vi "PathPlanner_Trajectory_ReadCSVFile.vi"(8 "error in (no error)":errorcluster, 11 "FileName":string="trajectory.csv") -> (0 "error out":errorcluster, 3 "outTRAJECTORY":T1 {"States"."TargetHolonomicRotation"."SIN" format="%13.4f"; "States"."TargetHolonomicRotation"."COS" format="%13.4f"; "States"."TargetHolonomicRotation"."VALUE" format="%13.4f"; "States"."Heading"."SIN" format="%13.4f"; "States"."Heading"."COS" format="%13.4f"; "States"."Heading"."VALUE" format="%13.4f"; "States"."PositionMeters"."Y" format="%14.3f"; "States"."PositionMeters"."X" format="%14.3f"}, 4 "Full FIlename":string)   [LabVIEW 2019, in "PathPlanner24.lvlib"]
doc: "Create a trajectory from a CSV file. This can be used on a PC or the RoboRIO. Normally the CSV file is created as output from one of the trajectory utility programs. The file could also be created manually or by a custom written program.\n\nParameters:\n - FileName -- Name of the CSV file to read. See file name notes for additional information.\n - Error In -- Input error cluster (optional)\n\nReturns:\n - outTrajectory - Trajectory data structure cluster\n - Error out - returned error cluster\n\nNotes on use:\n -- This routine writes informational messges to the console and to the driver station log.\n\nNotes on file naming:\n -- The file name must include the extention. \".csv\" is not automatically appended to the name. \n -- The file name can be a simple file or an absolute path. If a simple file name is used the default path on the RoboRIO is: \"home:\\lvuser\\natinst\\LabVIEW Data\". On a Windows PC the default path is the LabVIEW default directory. Normally this is: “%HOMEDRIVE%%HOMEPATH%\\Documents\\LabView Data\".\n -- Filenames on the RoboRIO, which runs Linux, are case sensitive.\n\nNotes on file contents:\n -- Blank lines are ignored.\n -- Lines that begin with either #, !, or ' in the first character are considered comments and are ignored. \n -- Other lines are interpretted as comma separated data as follows:\n -- Trajectory time -- seconds\n -- Expected velocity -- meters/sec\n -- Expected acceleration -- meters/sec^2\n -- Expected X position -- meters\n -- Expected Y position -- meters\n -- Expected heading (not necessarily robot orientation) -- radians\n -- Expected curvature (rotational portion of velocity) -- radians/meter\n -- Optional comment string. This ignored when reading file"
uses:
  PathPlanner24.lvlib
  <vilib>/Utility/error.llb/whitespace.ctl
  <vilib>/Rock Robotics/WPI/ThirdParty/JAS_Junk/TrajLib/TypeDef/TRANSLATION2D.ctl
  <vilib>/Rock Robotics/WPI/ThirdParty/JAS_Junk/TrajLib/Trajectory_Library.lvlib
  <vilib>/Rock Robotics/WPI/ThirdParty/JAS_Junk/TrajLib/TypeDef/ROTATION2D.ctl
  TypeDef/PathPlannerTrajectoryState.ctl
  TypeDef/PathPlannerConstraints.ctl
  TypeDef/PathPlannerTrajectory.ctl
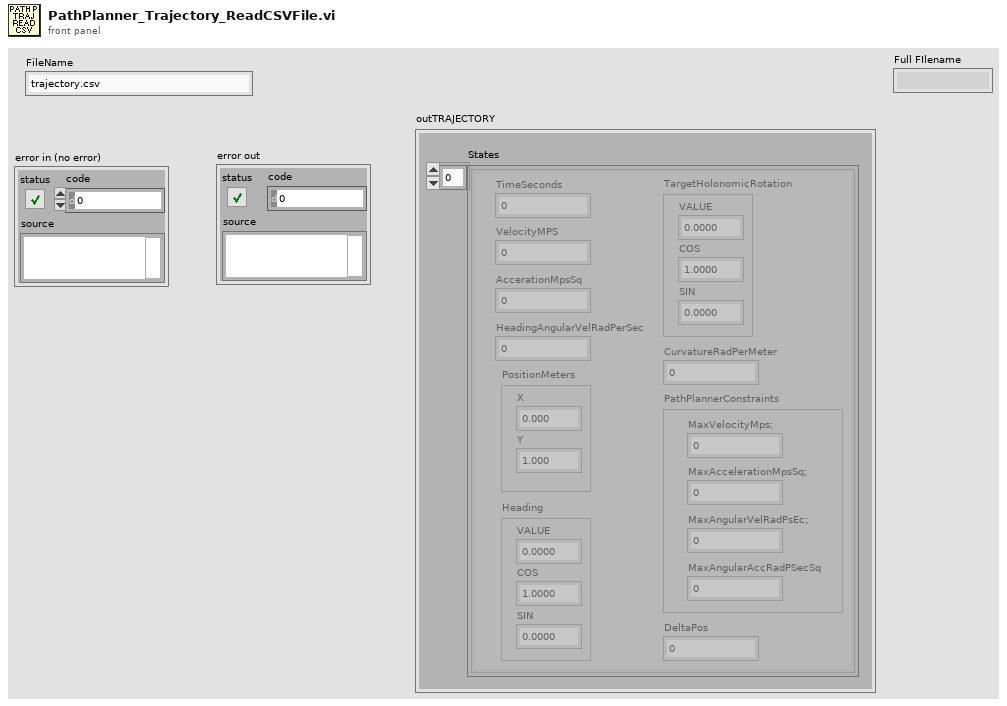
[diagram p1: front panel]
types:
  T1 = typedef "PathPlanner24.lvlib/PathPlannerTrajectory.ctl" = cluster{"States":T2[]}
  T2 = typedef "PathPlanner24.lvlib/PathPlannerTrajectoryState.ctl" = cluster{"TimeSeconds":dbl, "VelocityMPS":dbl, "AccerationMpsSq":dbl, "HeadingAngularVelRadPerSec":dbl, "PositionMeters":T3, "Heading":T4, "TargetHolonomicRotation":T4, "CurvatureRadPerMeter":dbl, "DeltaPos":dbl, "PathPlannerConstraints":T5}
  T3 = typedef "Trajectory_Library.lvlib/TRANSLATION2D.ctl" = cluster{"X":dbl, "Y":dbl}
  T4 = typedef "Trajectory_Library.lvlib/ROTATION2D.ctl" = cluster{"VALUE":dbl, "COS":dbl, "SIN":dbl}
  T5 = typedef "PathPlanner24.lvlib/PathPlannerConstraints.ctl" = cluster{"MaxVelocityMps;":dbl, "MaxAccelerationMpsSq;":dbl, "MaxAngularVelRadPsEc;":dbl, "MaxAngularAccRadPSecSq":dbl}
  T6 = enum16{"open", "replace", "create", "open or create", "replace or create", "replace or create with confirmation"}
  T7 = typedef "whitespace.ctl" = u16
  T8 = typedef "Trajectory_Library.lvlib/POSE2D.ctl" = cluster{"TRANSLATION":T3, "ROTATION":T4}
  T9 = typedef "PathPlanner24.lvlib/PathPlannerTrajectory.ctl" = cluster{"TotalTimeSeconds":dbl, "States":T2[]}
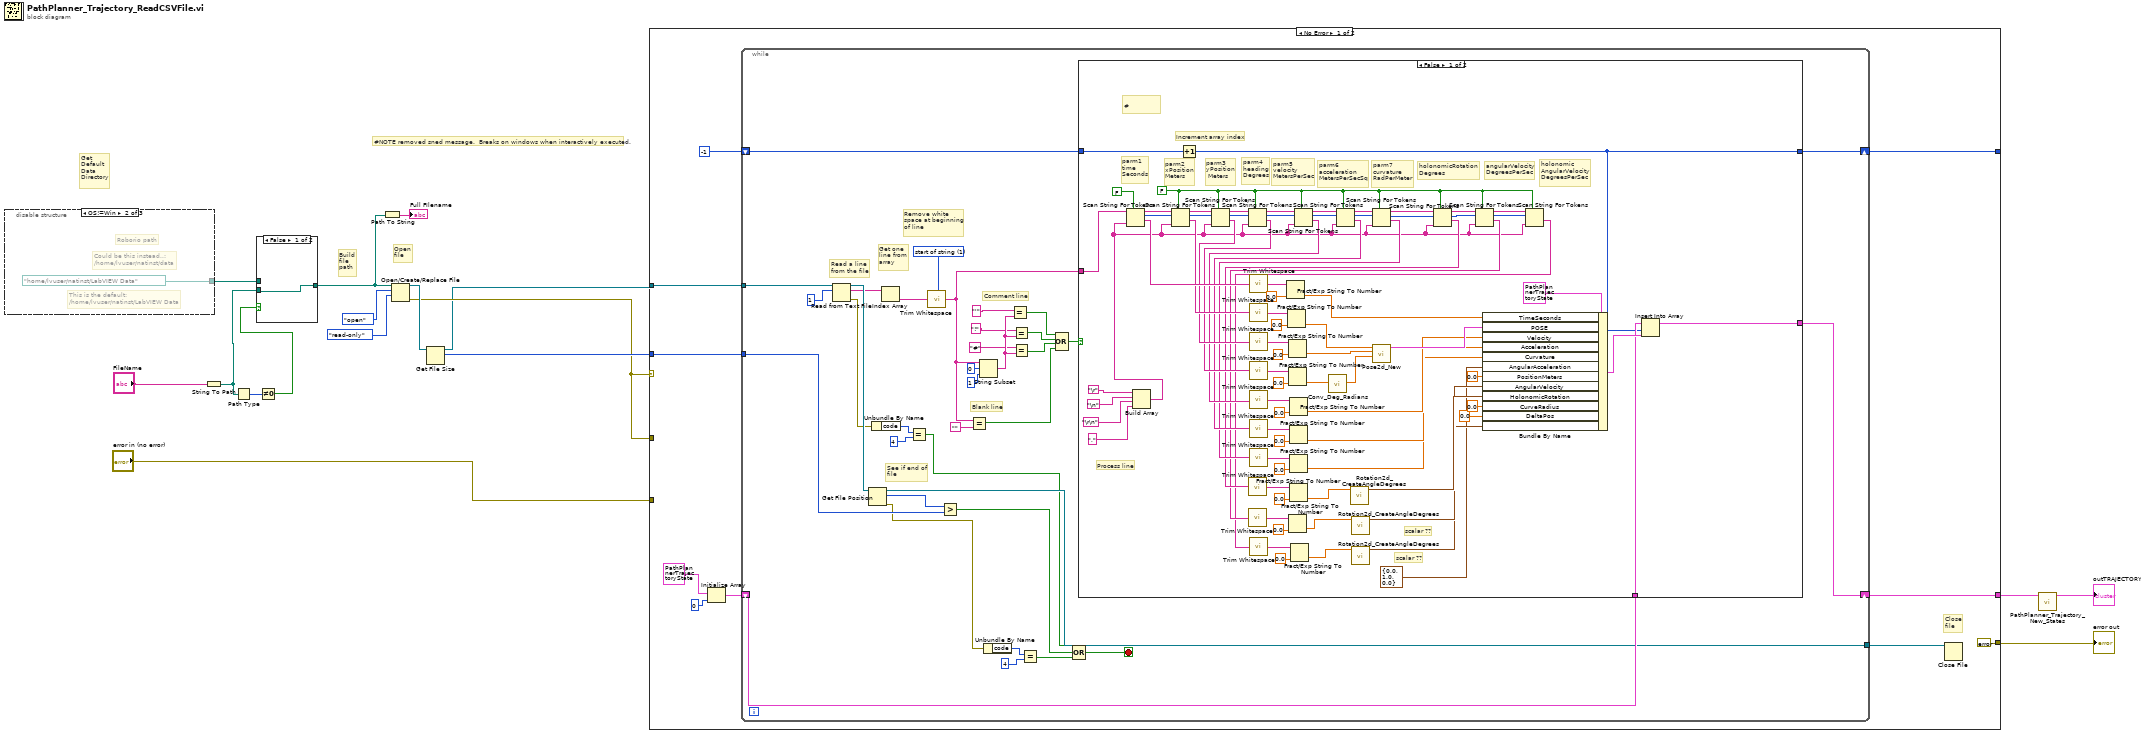
[diagram p0: block diagram]
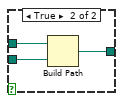
[diagram p2: hidden frame]
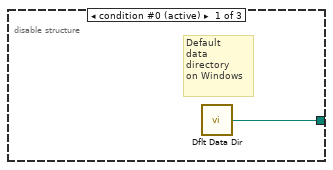
[diagram p3: hidden frame]
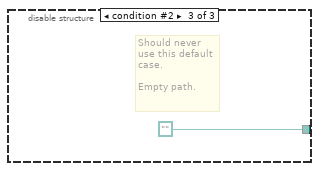
[diagram p4: hidden frame]
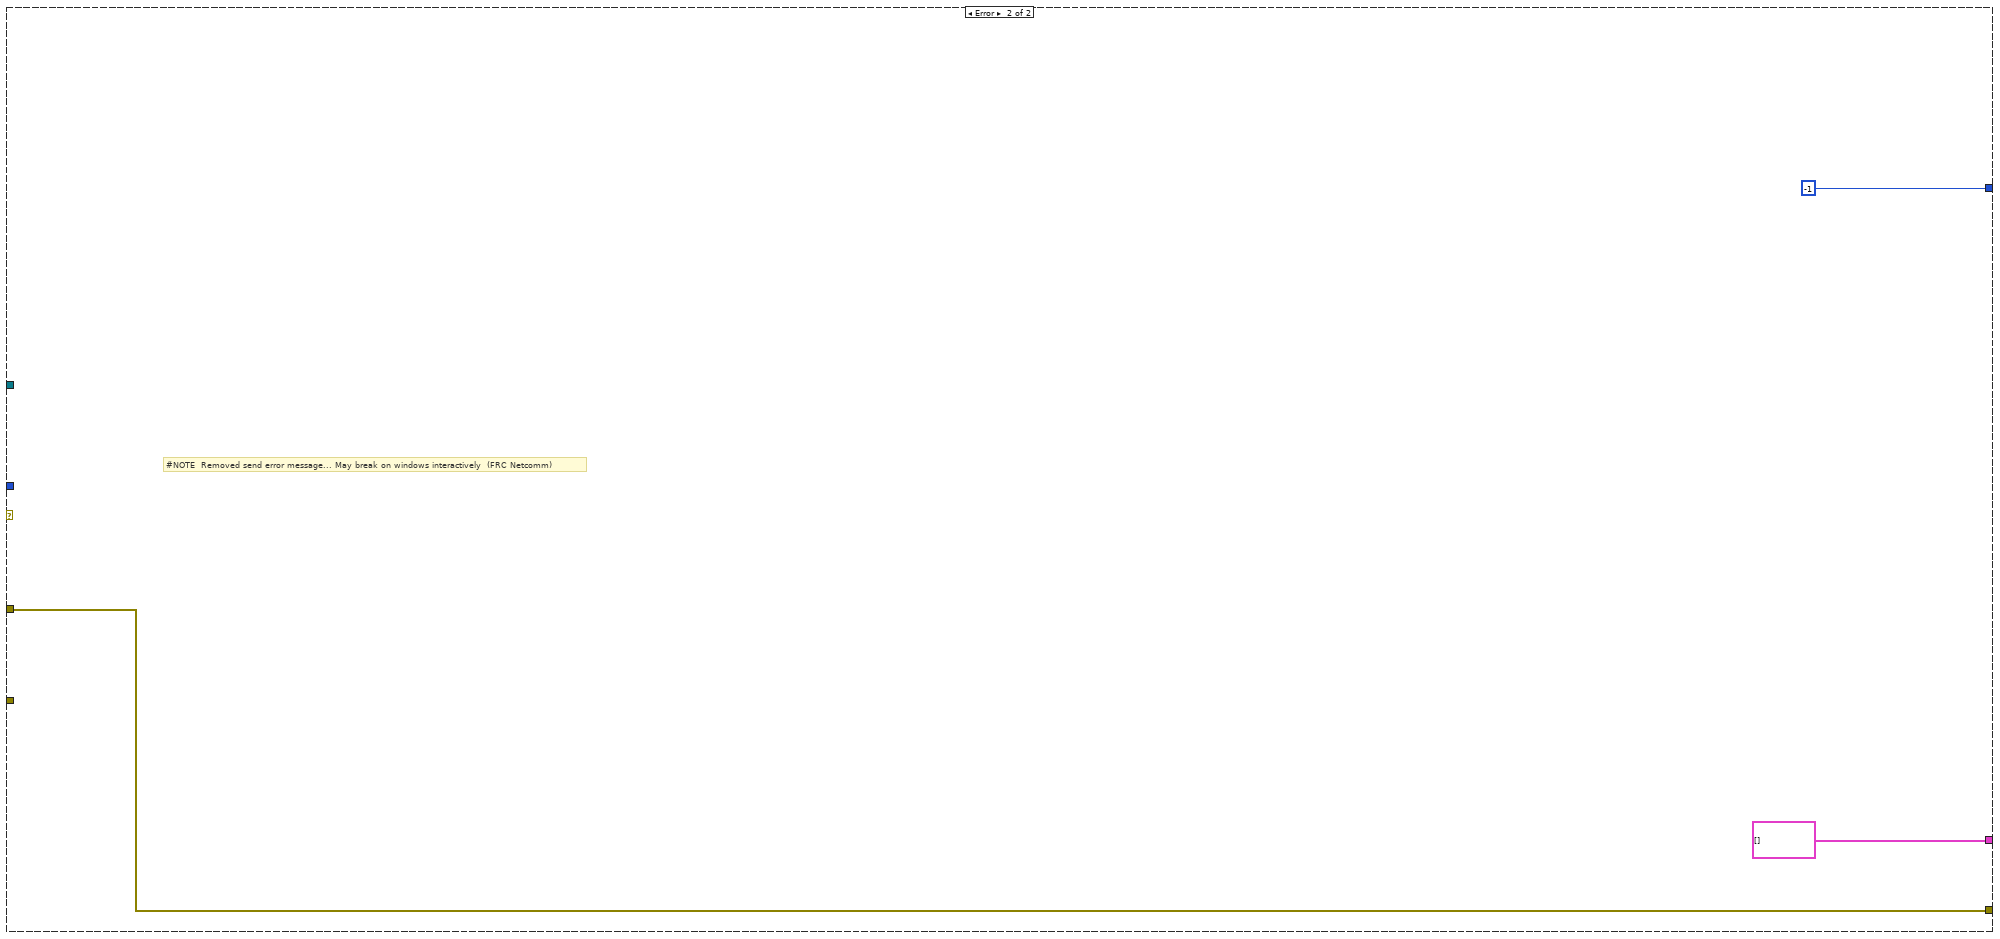
[diagram p6: hidden frame]
diagram:
  # "#NOTE removed sned message.  Breaks on windows when interactively executed."
  # "Get\nDefault\nData\nDirectory"
  # "Open\nfile"
  # "Build\nfile\npath"
  n1 = disable-structure shown="OS!=Win" {
    disable-tunnel: [w18 path "/home/lvuser/natinst/LabVIEW Data" path ""] -> w11
    frame condition #0 (active) {
      # "Default\ndata\ndirectory\non Windows"
      n2 = call <vilib>:"Dflt Data Dir.vi"() -> ("App:Default Data Directory"=w18:path)
    }
    frame condition #1 {
      # "This is the default:\n/home/lvuser/natinst/LabVIEW Data"
      # "Could be this instead..:\n/home/lvuser/natinst/data"
      # "Roborio path"
    }
    frame condition #2 {
      # "Should never\nuse this default\ncase.\n\nEmpty path."
    }
  }
  n3 = String To Path(string="FileName") -> (path=w8:path)
  n4 = Path Type(1:w8) -> (0:w7:i16)
  n5 = Not Equal To 0?(x=w7) -> (x != 0?=w6:bool)
  n6 = case shown="False" w6 {
    tunnel: [w21 w24] -> w14
    tunnel: w11 -> [_ w23]
    tunnel: w8 -> [w21 w22]
    frame False {
    }
    frame True {
      n7 = Build Path(base path=w23, name or relative path=w22) -> (appended path=w24:path)
    }
  }
  n8 = Path To String(path=w14) -> (string=→"Full FIlename":string)
  n9 = Open/Create/Replace File(file path (use dialog)=w14, operation (0:open)=T6."open", access (0:read/write)=enum16{"read/write", "read-only", "write-only"}."read-only") -> (refnum out=w15:refnum<file>, error out=w12:errorcluster)  [unwired: 3 in, 1 out]
  n10 = Get File Size(file=w15) -> (refnum out=w5:refnum<file>, size (in bytes)=w13:i64)  [unwired: 1 in, 1 out]
  n11 = case shown="No Error" w12 {
    tunnel: w5 -> [w34 _]
    tunnel: w13 -> [w32 _]
    tunnel: [w28 i16 -1] -> _
    tunnel: [w27 T2[] []] -> w2
    tunnel: w12 -> [_ w154]
    tunnel: [errorcluster {"status"=FALSE, "code"=0, "source"=""} ("error out") w154] -> w10
    tunnel: "error in (no error)" -> [_ _]
    frame No Error {
      # "Close\nfile"
      n12 = Initialize Array(T2 {"TimeSeconds"=0.0, "VelocityMPS"=0.0, "AccerationMpsSq"=0.0, "HeadingAngularVelRadPerSec"=0.0, "PositionMeters"={"X"=0.0, "Y"=1.0}, "Heading"={"VALUE"=0.0, "COS"=1.0, "SIN"=0.0}, "TargetHolonomicRotation"={"VALUE"=0.0, "COS"=1.0, "SIN"=0.0}, "CurvatureRadPerMeter"=0.0, "DeltaPos"=0.0, "PathPlannerConstraints"={"MaxVelocityMps;"=0.0, "MaxAccelerationMpsSq;"=0.0, "MaxAngularVelRadPsEc;"=0.0, "MaxAngularAccRadPSecSq"=0.0}} ("PathPlannerState"), 0 ("dimension size")) -> (w29:T2[])
      n13 = while {
        tunnel: w34 -> [w70]
        tunnel: w32 -> [w66]
        tunnel: [w46] -> w31
        shift-right: [w36] -> w28
        shift-left: i16 -1 -> [w50]
        shift-right: [w35] -> w27
        shift-left: w29 -> [w48]
        stop <- w44 stop-if-true
        w65 = T7 1 items=["both", "start of string", "end of string"] ("location (both)")
        # "Comment line"
        # "Blank line"
        # "Remove white \nspace at beginning\nof line"
        # "Get one\nline from\narray"
        # "Read a line\nfrom the file"
        # "See if end of \nfile"
        n14 = Read from Text File(file (use dialog)=w70, count=1) -> (refnum out=w68:refnum<file>, text=w64:string[], error out=w47:errorcluster)  [unwired: 2 in, 1 out]
        n15 = Get File Position(7:w68) -> (0:w39:errorcluster, 2:w67:i64, 3:w46:refnum<file>)  [unwired: 1 in]
        n16 = Unbundle By Name(w47) -> ("code"=w43:i32)
        n17 = Index Array(array=w64) -> (element=w63:string)  [unwired: 1 in]
        n18 = Equal?(x=w43, y=4) -> (x = y?=w38:bool)
        n19 = call <vilib>:"Trim Whitespace.vi"("string"=w63, "location (both)"=w65) -> ("trimmed string"=w49:string)
        n20 = Greater?(x=w67, y=w66) -> (0:w45:bool)
        n21 = Equal?(x=w49, y="") -> (x = y?=w52:bool)
        n22 = String Subset(string=w49, offset (0)=0, length (rest)=1 ("length (rest)")) -> (substring=w59:string)
        n23 = Unbundle By Name(w39) -> ("code"=w41:i32)
        n24 = Equal?(x="'", y=w59) -> (x = y?=w55:bool)
        n25 = Equal?(x="!", y=w59) -> (x = y?=w54:bool)
        n26 = Equal?(x="#", y=w59) -> (x = y?=w53:bool)
        n27 = Equal?(x=w41, y=4) -> (x = y?=w37:bool)
        n28 = Compound Arithmetic op=OR(w55, w54, w53, w52) -> (w51:bool)
        n29 = Compound Arithmetic op=OR(w38, w45, w37) -> (w44:bool)
        n30 = case shown="False" w51 {
          tunnel: w50 -> [w151 w152]
          tunnel: [w116 w152] -> w36
          tunnel: w49 -> [w115 _]
          tunnel: w48 -> [w118 w153]
          tunnel: [w117 w153] -> w35
          frame False {
            w97 = FALSE ("allow empty tokens? (F)")
            # "scalar ??"
            # "scalar ??"
            # "holonomic\nAngularVelocity\nDegreesPerSec"
            # "angularVelocity\nDegreesPerSec"
            # "holonomicRotation\nDegrees"
            # "#"
            # "parm6\nacceleration\nMetersPerSecSq"
            # "parm7\ncurvature\nRadPerMeter"
            # "parm5\nvelocity\nMetersPerSec"
            # "parm4\nheading\nDegrees"
            # "parm3\nyPosition\n Meters"
            # "parm2\nxPosition\nMeters"
            # "parm1\ntime\nSeconds"
            # "Increment array index"
            # "Process line"
            n31 = Build Array("\r", "\n", "\r\n", ",") -> (w75:string[])
            n32 = Scan String For Tokens(5:FALSE ("allow empty tokens? (F)"), 6:w75, 9:w115) -> (1:w135:string, 2:w140:i32, 3:w145:string)  [unwired: 3 in, 1 out]
            n33 = Scan String For Tokens(5:w97, 6:w75, 8:w140, 9:w145) -> (1:w134:string, 2:w139:i32, 3:w144:string)  [unwired: 2 in, 1 out]
            n34 = Increment(x=w151) -> (x+1=w116:i16)
            n35 = Scan String For Tokens(5:w97, 6:w75, 8:w139, 9:w144) -> (1:w133:string, 2:w138:i32, 3:w143:string)  [unwired: 2 in, 1 out]
            n36 = Scan String For Tokens(5:w97, 6:w75, 8:w138, 9:w143) -> (1:w132:string, 2:w137:i32, 3:w142:string)  [unwired: 2 in, 1 out]
            n37 = call <vilib>:"Trim Whitespace.vi"("string"=w135) -> ("trimmed string"=w106:string)  [unwired: 1 in]
            n38 = call <vilib>:"Trim Whitespace.vi"("string"=w134) -> ("trimmed string"=w128:string)  [unwired: 1 in]
            n39 = call <vilib>:"Trim Whitespace.vi"("string"=w133) -> ("trimmed string"=w123:string)  [unwired: 1 in]
            n40 = call <vilib>:"Trim Whitespace.vi"("string"=w132) -> ("trimmed string"=w122:string)  [unwired: 1 in]
            n41 = Fract/Exp String To Number(string=w106, default (0 dbl)=0.0 ("default (0 DBL)")) -> (number=w107:dbl)  [unwired: 2 in, 1 out]
            n42 = Fract/Exp String To Number(string=w128, default (0 dbl)=0.0 ("default (0 DBL)")) -> (number=w104:dbl)  [unwired: 2 in, 1 out]
            n43 = Fract/Exp String To Number(string=w123, default (0 dbl)=0.0 ("default (0 DBL)")) -> (number=w103:dbl)  [unwired: 2 in, 1 out]
            n44 = Fract/Exp String To Number(string=w122, default (0 dbl)=0.0 ("default (0 DBL)")) -> (number=w102:dbl)  [unwired: 2 in, 1 out]
            n45 = Scan String For Tokens(5:w97, 6:w75, 8:w137, 9:w142) -> (1:w131:string, 2:w136:i32, 3:w141:string)  [unwired: 2 in, 1 out]
            n46 = call <vilib>:"Trim Whitespace.vi"("string"=w131) -> ("trimmed string"=w121:string)  [unwired: 1 in]
            n47 = Fract/Exp String To Number(string=w121, default (0 dbl)=0.0 ("default (0 DBL)")) -> (number=w100:dbl)  [unwired: 2 in, 1 out]
            n48 = call <vilib>:"Conv_Deg_Radians.vi"("Degress"=w102) -> ("Radians"=w101:dbl)  [unwired: 10 in]
            n49 = Scan String For Tokens(5:w97, 6:w75, 8:w136, 9:w141) -> (1:w130:string, 2:w109:i32, 3:w110:string)  [unwired: 2 in, 1 out]
            n50 = call <vilib>:"Trim Whitespace.vi"("string"=w130) -> ("trimmed string"=w120:string)  [unwired: 1 in]
            n51 = Fract/Exp String To Number(string=w120, default (0 dbl)=0.0 ("default (0 DBL)")) -> (number=w99:dbl)  [unwired: 2 in, 1 out]
            n52 = Scan String For Tokens(5:w97, 6:w75, 8:w109, 9:w110) -> (1:w108:string, 2:w93:i32, 3:w96:string)  [unwired: 2 in, 1 out]
            n53 = call <vilib>:"Trim Whitespace.vi"("string"=w108) -> ("trimmed string"=w111:string)  [unwired: 1 in]
            n54 = Fract/Exp String To Number(string=w111, default (0 dbl)=0.0 ("default (0 DBL)")) -> (number=w98:dbl)  [unwired: 2 in, 1 out]
            n55 = call <vilib>:"Pose2d_New.vi"("Heading"=w101, "Y"=w103, "X"=w104) -> ("out POSe"=w113:T8)  [unwired: 8 in]
            n56 = Scan String For Tokens(5:w97, 6:w75, 8:w93, 9:w96) -> (1:w84:string, 2:w92:i32, 3:w95:string)  [unwired: 2 in, 1 out]
            n57 = call <vilib>:"Trim Whitespace.vi"("string"=w84) -> ("trimmed string"=w89:string)  [unwired: 1 in]
            n58 = Fract/Exp String To Number(string=w89, default (0 dbl)=0.0 ("default (0 DBL)")) -> (number=w83:dbl)  [unwired: 2 in, 1 out]
            n59 = call <vilib>:"Rotation2d_CreateAngleDegrees.vi"("Angle_Degrees"=w83) -> ("ROTATION"=w82:T4)  [unwired: 10 in]
            n60 = Scan String For Tokens(5:w97, 6:w75, 8:w92, 9:w95) -> (1:w81:string, 2:w91:i32, 3:w94:string)  [unwired: 2 in, 1 out]
            n61 = call <vilib>:"Trim Whitespace.vi"("string"=w81) -> ("trimmed string"=w87:string)  [unwired: 1 in]
            n62 = Fract/Exp String To Number(string=w87, default (0 dbl)=0.0 ("default (0 DBL)")) -> (number=w80:dbl)  [unwired: 2 in, 1 out]
            n63 = call <vilib>:"Rotation2d_CreateAngleDegrees.vi"("Angle_Degrees"=w80) -> ("ROTATION"=w79:T4)  [unwired: 10 in]
            n64 = Scan String For Tokens(5:w97, 6:w75, 8:w91, 9:w94) -> (1:w76:string)  [unwired: 2 in, 3 out]
            n65 = call <vilib>:"Trim Whitespace.vi"("string"=w76) -> ("trimmed string"=w85:string)  [unwired: 1 in]
            n66 = Fract/Exp String To Number(string=w85, default (0 dbl)=0.0 ("default (0 DBL)")) -> (number=w78:dbl)  [unwired: 2 in, 1 out]
            n67 = call <vilib>:"Rotation2d_CreateAngleDegrees.vi"("Angle_Degrees"=w78) -> ("ROTATION"=w77:T4)  [unwired: 10 in]
            n68 = Bundle By Name(cluster=T2 {"TimeSeconds"=0.0, "VelocityMPS"=0.0, "AccerationMpsSq"=0.0, "HeadingAngularVelRadPerSec"=0.0, "PositionMeters"={"X"=0.0, "Y"=1.0}, "Heading"={"VALUE"=0.0, "COS"=1.0, "SIN"=0.0}, "TargetHolonomicRotation"={"VALUE"=0.0, "COS"=1.0, "SIN"=0.0}, "CurvatureRadPerMeter"=0.0, "DeltaPos"=0.0, "PathPlannerConstraints"={"MaxVelocityMps;"=0.0, "MaxAccelerationMpsSq;"=0.0, "MaxAngularVelRadPsEc;"=0.0, "MaxAngularAccRadPSecSq"=0.0}} ("PathPlannerState"), "TimeSeconds"=w107, "POSE"=w113, "Velocity"=w100, "Acceleration"=w99, "Curvature"=w98, "AngularAcceleration"=T4 {"VALUE"=0.0, "COS"=1.0, "SIN"=0.0}, "PositionMeters"=0.0, "AngularVelocity"=w79, "HolonomicRotation"=w82, "CurveRadius"=0.0, "DeltaPos"=0.0, "HolonomicAngular\nvelocity Deg/Sec"=w77) -> (w119:T2)
            n69 = Insert Into Array(array=w118, index=w116, new element=w119) -> (w117:T2[])
          }
          frame True {
            # "Comment -- ignore."
          }
        }
      }
      n70 = Close File(refnum=w31) -> ()  [unwired: 1 in, 2 out]
    }
    frame Error {
      # "#NOTE  Removed send error message... May break on windows interactively  (FRC Netcomm)"
    }
  }
  "error out" <- w10
  n71 = call "PathPlanner_Trajectory_New_States.vi"("PathPlannerStates"=w2) -> ("PathPlannerTrajectory"=→"outTRAJECTORY":T9)  [unwired: 10 in]
